vi "Find Tests In Suite.vi"(8 "error in (no error)":errorcluster, 10 "Test Suite":refnum<class "LUnit Test Suite.lvclass">, 11 "Test Finder In":refnum<class "Test Finder.lvclass">) -> (0 "error out":errorcluster, 3 "Test Finder Out":refnum<class "Test Finder.lvclass">)   [LabVIEW 2020, in "Test Finder.lvclass"]
uses:
  Test Finder.lvclass
  Test Suite/LUnit Test Suite.lvclass
  Test Suite/LUnit Test Suite.lvclass/LUnit Test Suite.ctl
  Test Case/LUnit Test Case.lvclass
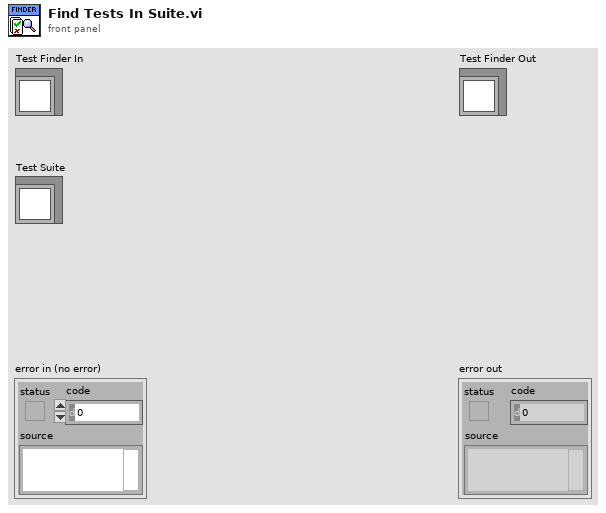
[diagram p1: front panel]
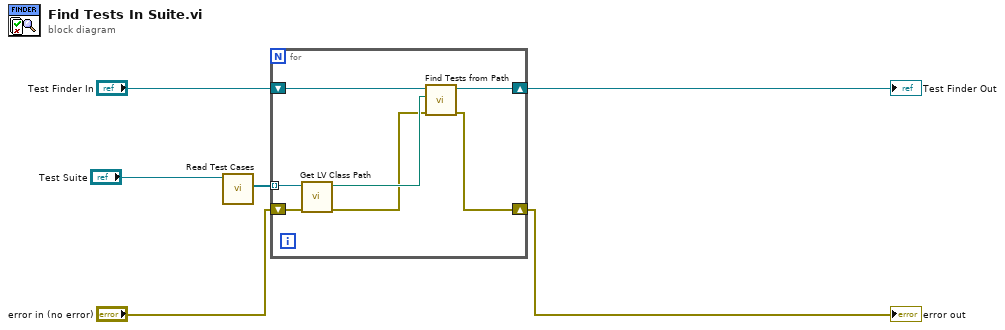
[diagram p0: block diagram]
diagram:
  n1 = call "Read Test Cases.vi"("Test Suite In"="Test Suite") -> ("Test Cases"=w5:refnum<class "LUnit Test Case.lvclass">[])  [unwired: 9 in, 1 out]
  n2 = for {
    tunnel: w5 -> [w13] mode=indexing
    shift-right: [w8] -> w1
    shift-left: "error in (no error)" -> [w12]
    shift-right: [w9] -> w2
    shift-left: "Test Finder In" -> [w11]
    n3 = call <vilib>:"Get LV Class Path.vi"("error in (no error)"=w12, "object"=w13) -> ("error out"=w7:errorcluster, "class path"=w10:path)  [unwired: 8 in]
    n4 = call-dynamic "Find Tests from Path.vi"("error in (no error)"=w7, "Project or Class Path"=w10, "Test Case Finder In"=w11) -> ("error out"=w8:errorcluster, "Test Case Finder Out"=w9:refnum<class "Test Finder.lvclass">)  [unwired: 7 in]
  }
  "error out" <- w1
  "Test Finder Out" <- w2
